vi "3_2.vi"() -> ()   [LabVIEW 2019]
panel:
  in  "Stop":bool
  out "X(i-3)":i32
  out "X(i-2)":i32
  out "X(i-1)":i32
  out "X(i)":i32
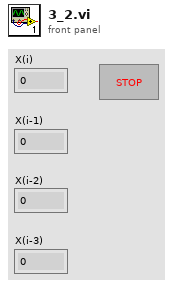
[diagram p1: front panel]
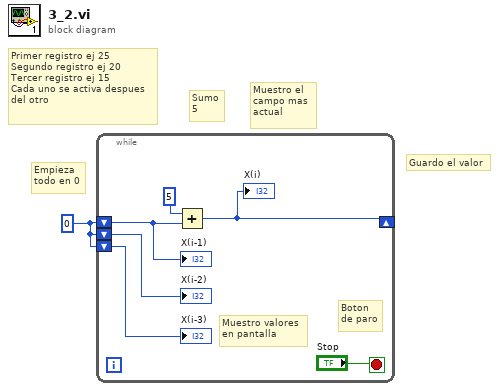
[diagram p0: block diagram]
diagram:
  w1 = 0
  # "Primer registro ej 25\nSegundo registro ej 20\nTercer registro ej 15\nCada uno se activa despues\ndel otro"
  # "Guardo el valor"
  # "Muestro el \ncampo mas\nactual"
  # "Sumo\n5"
  # "Empieza \ntodo en 0"
  n1 = while {
    shift-right: [w5] -> _
    shift-left: w1 -> [w4]
    shift-left: w1 -> [w3]
    shift-left: w1 -> [w2]
    stop <- "Stop" stop-if-true
    # "Boton\nde paro"
    # "Muestro valores\nen pantalla"
    n2 = Add(x=5, y=w4) -> (x+y=w5:i32)
    "X(i)" <- w5
    "X(i-1)" <- w4
    "X(i-2)" <- w3
    "X(i-3)" <- w2
  }
